vi "Vision_Processing_L_R6.vi"(0 "Current State":T2(ring), 1 "Image Dst":T7=refnum, 2 "Inpute Image":T7=refnum, 3 "Startup Flag":bool, 5 "Current ROI Descriptor":T12={"Global Rectangle"=[81, 70, 256, 199], "Contours"=[{"ID"=enum."External", "Type"=12, "Coordinates"=[81, 70, 256, 199, 0]}]} {"Contours"."Type" items=["No Selection", "Point", "Line", "Rectangle", "Oval", "Polygon", "Freehand Region", "Annulus", "Unused2", "Unused3", "Broken Line", "Freehand Line", "Rotated Rectangle"]}, 7 "error in (no error)":errorcluster, 8 "Current Settings":T10={"Curve Parameters"={"Extraction Mode"=1, "Edge Threshold"=150, "Edge Filter Size"=0, "Min Length"=25, "Row Search Step Size"=15, "Col Search Step Size"=15, "Max Endpoint Gap"=2, "Closed"=TRUE, "Subpixel"=TRUE}, "Match Mode"={"Rotation"=TRUE, "Scale"=TRUE, "Occlusion"=TRUE, "Reserved"=FALSE, "Reserved"=FALSE, "Reserved"=FALSE}, "Range Settings"=[{"Match Constraints"=0, "Min"=-5.0, "Max"=5.0}, {"Match Constraints"=1, "Min"=90.5926284790039, "Max"=120.5926284790039}, {"Match Constraints"=2, "Min"=0.0, "Max"=25.0}], "Number of Matches"=1, "Minimum Match Score"=866.6676, "SubPixel Accuracy"=TRUE, "Adv. Geometric Match Options 2"=[{"Setup Data Item"=20, "Item Value"=0.0}, {"Setup Data Item"=22, "Item Value"=1.0}]} {"Curve Parameters"."Extraction Mode" items=["Normal", "Uniform Regions"]; "Curve Parameters"."Edge Filter Size" items=["Fine", "Normal", "Contour Tracing"]; "Curve Parameters"."Max Endpoint Gap" min=0; "Curve Parameters"."Col Search Step Size" min=1 max=255 step=1; "Curve Parameters"."Row Search Step Size" min=1 max=255 step=1; "Curve Parameters"."Min Length" min=0; "Curve Parameters"."Edge Threshold" min=1 max=350 step=1; "Range Settings"."Max" format="%.2f"; "Range Settings"."Min" format="%.2f"; "Range Settings"."Match Constraints" items=["Rotation Angle (degrees)", "Scale Factor (%)", "Occlusion (%)"]; "Adv. Geometric Match Options 2"."Setup Data Item" items=["Curve Extraction Mode", "Curve Edge Threshold", "Curve Edge Filter Size", "Min Curve Length", "Curve Row Search Step Size", "Curve Col Search Step Size", "Curve Max Endpoint Gap", "Extract Closed Curves", "Enable Subpixel Curve Extraction", "Enable Correlation Score", "Enable Subpixel Accuracy", "Subpixel Iterations", "Subpixel Tolerance", "Initial Match List Length", "Enable Target Template Curve Score", "Min Match Separation Distance", "Min Match Separation Angle", "Min Match Separation Scale", "Max Match Overlap", "Enable Coarse Result", "Enable Calibration Support", "Enable Contrast Reversal", "Search Strategy", "Refinement Match Factor", "Subpixel Match Factor"]}, 9 "Sub Beacon Search Enable":bool[](array[boolean])=[FALSE, FALSE, FALSE, FALSE, FALSE], 10 "History Data - IN":T6={"Valid Beacon History - in"=[TRUE, TRUE, TRUE, TRUE, TRUE, TRUE, TRUE, TRUE, TRUE, TRUE, TRUE, TRUE, TRUE, TRUE, TRUE, TRUE, TRUE, TRUE, TRUE, TRUE], "Valid Score History"=[1000.0, 989.88427734375, 989.88427734375, 989.88427734375, 988.6851196289062, 989.88427734375, 989.0393676757812, 988.6851196289062, 989.88427734375, 987.4860229492188, 989.88427734375, 992.1041870117188, 989.3124389648438, 990.905029296875, 990.5115356445312, 992.1041870117188, 992.1041870117188, 989.88427734375, 991.870361328125, 987.4860229492188], "Valid Scale History"=[103.47016143798828, 106.12324523925781, 106.12324523925781, 106.12324523925781, 106.12324523925781, 106.12324523925781, 106.12324523925781, 106.12324523925781, 106.12324523925781, 106.12324523925781, 106.12324523925781, 105.79054260253906, 106.12324523925781, 105.71609497070312, 106.04004669189453, 105.79054260253906, 105.79054260253906, 106.12324523925781, 105.74315643310547, 106.12324523925781]} {"Valid Scale History" format="%#_13g"; "Valid Score History" format="%#_13g"}, 13 "Last Averages":T1={"Avg Scale - Last"=105.5926284790039, "Avg Score - Last"=991.6675903320313}, 16 "History Size":i32=10, 26 "State Count - in":i32) -> (4 "State Count - out":i32=1, 11 "Avg Scale":dbl=105.5926284790039, 12 "Avg Score":dbl=991.6675903320313, 14 "Tracking Info":T3={"Tracking Coordinates"={"X"=168.53689575195312, "Y"=129.63653564453125}, "Current Valid"=TRUE, "Current State - Out"=enum."Sub - 2"}, 15 "Next Main ROI Descriptor":T4={"Global Rectangle"=[81, 70, 256, 199], "Contours"=[{"ID"=enum."External", "Type"=12, "Coordinates"=[81, 70, 256, 199, 0]}]} {"Contours"."Type" items=["No Selection", "Point", "Line", "Rectangle", "Oval", "Polygon", "Freehand Region", "Annulus", "Unused2", "Unused3", "Broken Line", "Freehand Line", "Rotated Rectangle"]}, 17 "Beacon - Scales":sgl[](array[numeric])=[97.53761, 105.154755, 0.0, 0.0, 0.0], 18 "History Data - Out":T5={"Valid Beacon History\nOut"=[TRUE, TRUE, TRUE, TRUE, TRUE, TRUE, TRUE, TRUE, TRUE, TRUE, TRUE, TRUE, TRUE, TRUE, TRUE, TRUE, TRUE, TRUE, TRUE, TRUE], "Valid Score History\nOut"=[1000.0, 989.88427734375, 989.88427734375, 989.88427734375, 988.6851196289062, 989.88427734375, 989.0393676757812, 988.6851196289062, 989.88427734375, 987.4860229492188, 989.88427734375, 992.1041870117188, 989.3124389648438, 990.905029296875, 990.5115356445312, 992.1041870117188, 992.1041870117188, 989.88427734375, 991.870361328125, 987.4860229492188], "Valid Scale History\nOut"=[103.47016143798828, 106.12324523925781, 106.12324523925781, 106.12324523925781, 106.12324523925781, 106.12324523925781, 106.12324523925781, 106.12324523925781, 106.12324523925781, 106.12324523925781, 106.12324523925781, 105.79054260253906, 106.12324523925781, 105.71609497070312, 106.04004669189453, 105.79054260253906, 105.79054260253906, 106.12324523925781, 105.74315643310547, 106.12324523925781]} {"Valid Scale History\nOut" format="%#_13g"; "Valid Score History\nOut" format="%#_13g"}, 19 "Y Coordinates":sgl[](array[numeric])=[137.61583, 129.42519, 0.0, 0.0, 0.0], 20 "Beacons Found":bool[](array[boolean])=[TRUE, TRUE, FALSE, FALSE, FALSE], 21 "X Coordinates":sgl[](array[numeric])=[137.6292, 203.13261, 0.0, 0.0, 0.0], 22 "Next State":T2(ring), 23 "Lock Status":bool=TRUE, 24 "Startup Flag - out":bool, 25 "New Settings":T10={"Curve Parameters"={"Extraction Mode"=1, "Edge Threshold"=150, "Edge Filter Size"=0, "Min Length"=25, "Row Search Step Size"=15, "Col Search Step Size"=15, "Max Endpoint Gap"=2, "Closed"=TRUE, "Subpixel"=TRUE}, "Match Mode"={"Rotation"=TRUE, "Scale"=TRUE, "Occlusion"=TRUE, "Reserved"=FALSE, "Reserved"=FALSE, "Reserved"=FALSE}, "Range Settings"=[{"Match Constraints"=0, "Min"=-5.0, "Max"=5.0}, {"Match Constraints"=1, "Min"=90.5926284790039, "Max"=120.5926284790039}, {"Match Constraints"=2, "Min"=0.0, "Max"=25.0}], "Number of Matches"=1, "Minimum Match Score"=866.6676, "SubPixel Accuracy"=TRUE, "Adv. Geometric Match Options 2"=[{"Setup Data Item"=20, "Item Value"=0.0}, {"Setup Data Item"=22, "Item Value"=1.0}]} {"Curve Parameters"."Extraction Mode" items=["Normal", "Uniform Regions"]; "Curve Parameters"."Edge Filter Size" items=["Fine", "Normal", "Contour Tracing"]; "Curve Parameters"."Max Endpoint Gap" min=0; "Curve Parameters"."Col Search Step Size" min=1 max=255 step=1; "Curve Parameters"."Row Search Step Size" min=1 max=255 step=1; "Curve Parameters"."Min Length" min=0; "Curve Parameters"."Edge Threshold" min=1 max=350 step=1; "Range Settings"."Max" format="%.2f"; "Range Settings"."Min" format="%.2f"; "Range Settings"."Match Constraints" items=["Rotation Angle (degrees)", "Scale Factor (%)", "Occlusion (%)"]}, 27 "Right Image 2":T7(plugin-control))   [LabVIEW 2015]
uses:
  <vilib>/vision/Image Controls.llb/IMAQ Image.ctl
  <vilib>/vision/Pattern Matching.llb/IMAQ Curve Parameters.ctl
  <vilib>/vision/Pattern Matching.llb/IMAQ Match Range Setting.ctl
panel:
  in  "Sub - 4 - FIle Path":path=path "/home/lvuser/natinst/bin/BeaconTemplates/4_beacons_left.png"
  in  "3 / 2\nTransition Scale":sgl=100.0
  in  "Score\nCushion- tight":dbl=75.0
  in  "Main ROI Decay\nper Fail (Vertical)":i32=5
  in  "ROI_factor(Horiztonal) SCR":sgl=1.7
  in  "ROI_factor(vertical) SCR":sgl=1.5
  in  "Sub - 2 File Path":path=path "/home/lvuser/natinst/bin/BeaconTemplates/2_beacons_left.png"
  in  "Scale Decay \nFactor":dbl=0.5
  in  "Scale Decay \nFactor":dbl=5.0
  in  "Valid Treshold\nfor Lock":i16=3
  in  "Horiztonall Beacon \nCushion (pixels)":sgl=25.0
  out "New Min Score":dbl=866.6675903320313
  out "New Low Scale":dbl=90.5926284790039
  out "New high Scale":dbl=120.5926284790039
  in  "Absolute\nMinimum Score":dbl=700.0
  in  "Absolute\nMaximum Scale":dbl=300.0
  in  "Absolute\nMinimum Scale":dbl=10.0
  in  "Default No Lock\nSetting Values":T11={"Min Scale"=20.0, "Max Scale"=170.0, "Min Score"=800.0}
  in  "Score\nCushion":dbl=125.0
  in  "Scale \nCushion":dbl=15.0
  in  "5 / 4\nTransition Scale":sgl=78.0
  in  "4 / 3\nTransition Scale":sgl=85.0
  in  "Timeout \nThrehsold":i32=1000
  in  "Main ROI Decay\nper Fail (Horiztonal)":i32=25
  in  "ROI_factor(Horiztonal) LR":sgl=5.0
  in  "ROI_factor(vertical) LR":sgl=1.5
  in  "ROI_factor(vertical) SR":sgl=2.7
  in  "ROI_factor(Horiztonal) SR":sgl=2.0
  out "Current  Score":sgl=1000.0
  out "Current  Scale":sgl=103.47016
  in  "Fail Count - In":i32
  in  "Sub Beacon Template File Path - ARRAY":path[](array[path])=[path "/home/lvuser/natinst/bin/BeaconTemplates/Sub1.png", path "/home/lvuser/natinst/bin/BeaconTemplates/Sub2.png", path "/home/lvuser/natinst/bin/BeaconTemplates/Sub3.png", path "/home/lvuser/natinst/bin/BeaconTemplates/Sub4.png", path "/home/lvuser/natinst/bin/BeaconTemplates/Sub5.png"]
  in  "Sub - 3 - FIle Path":path=path "/home/lvuser/natinst/bin/BeaconTemplates/3_beacons_left.png"
  in  "Normal - 5 - File Path":path=path "/home/lvuser/natinst/bin/BeaconTemplates/5_beacons.png"
  # "INPUTS"
  # "FILE PATHS"
  # "CONFIG"
  # "OUTPUTS"
  # "************"
  # "Range"
  # "Range"
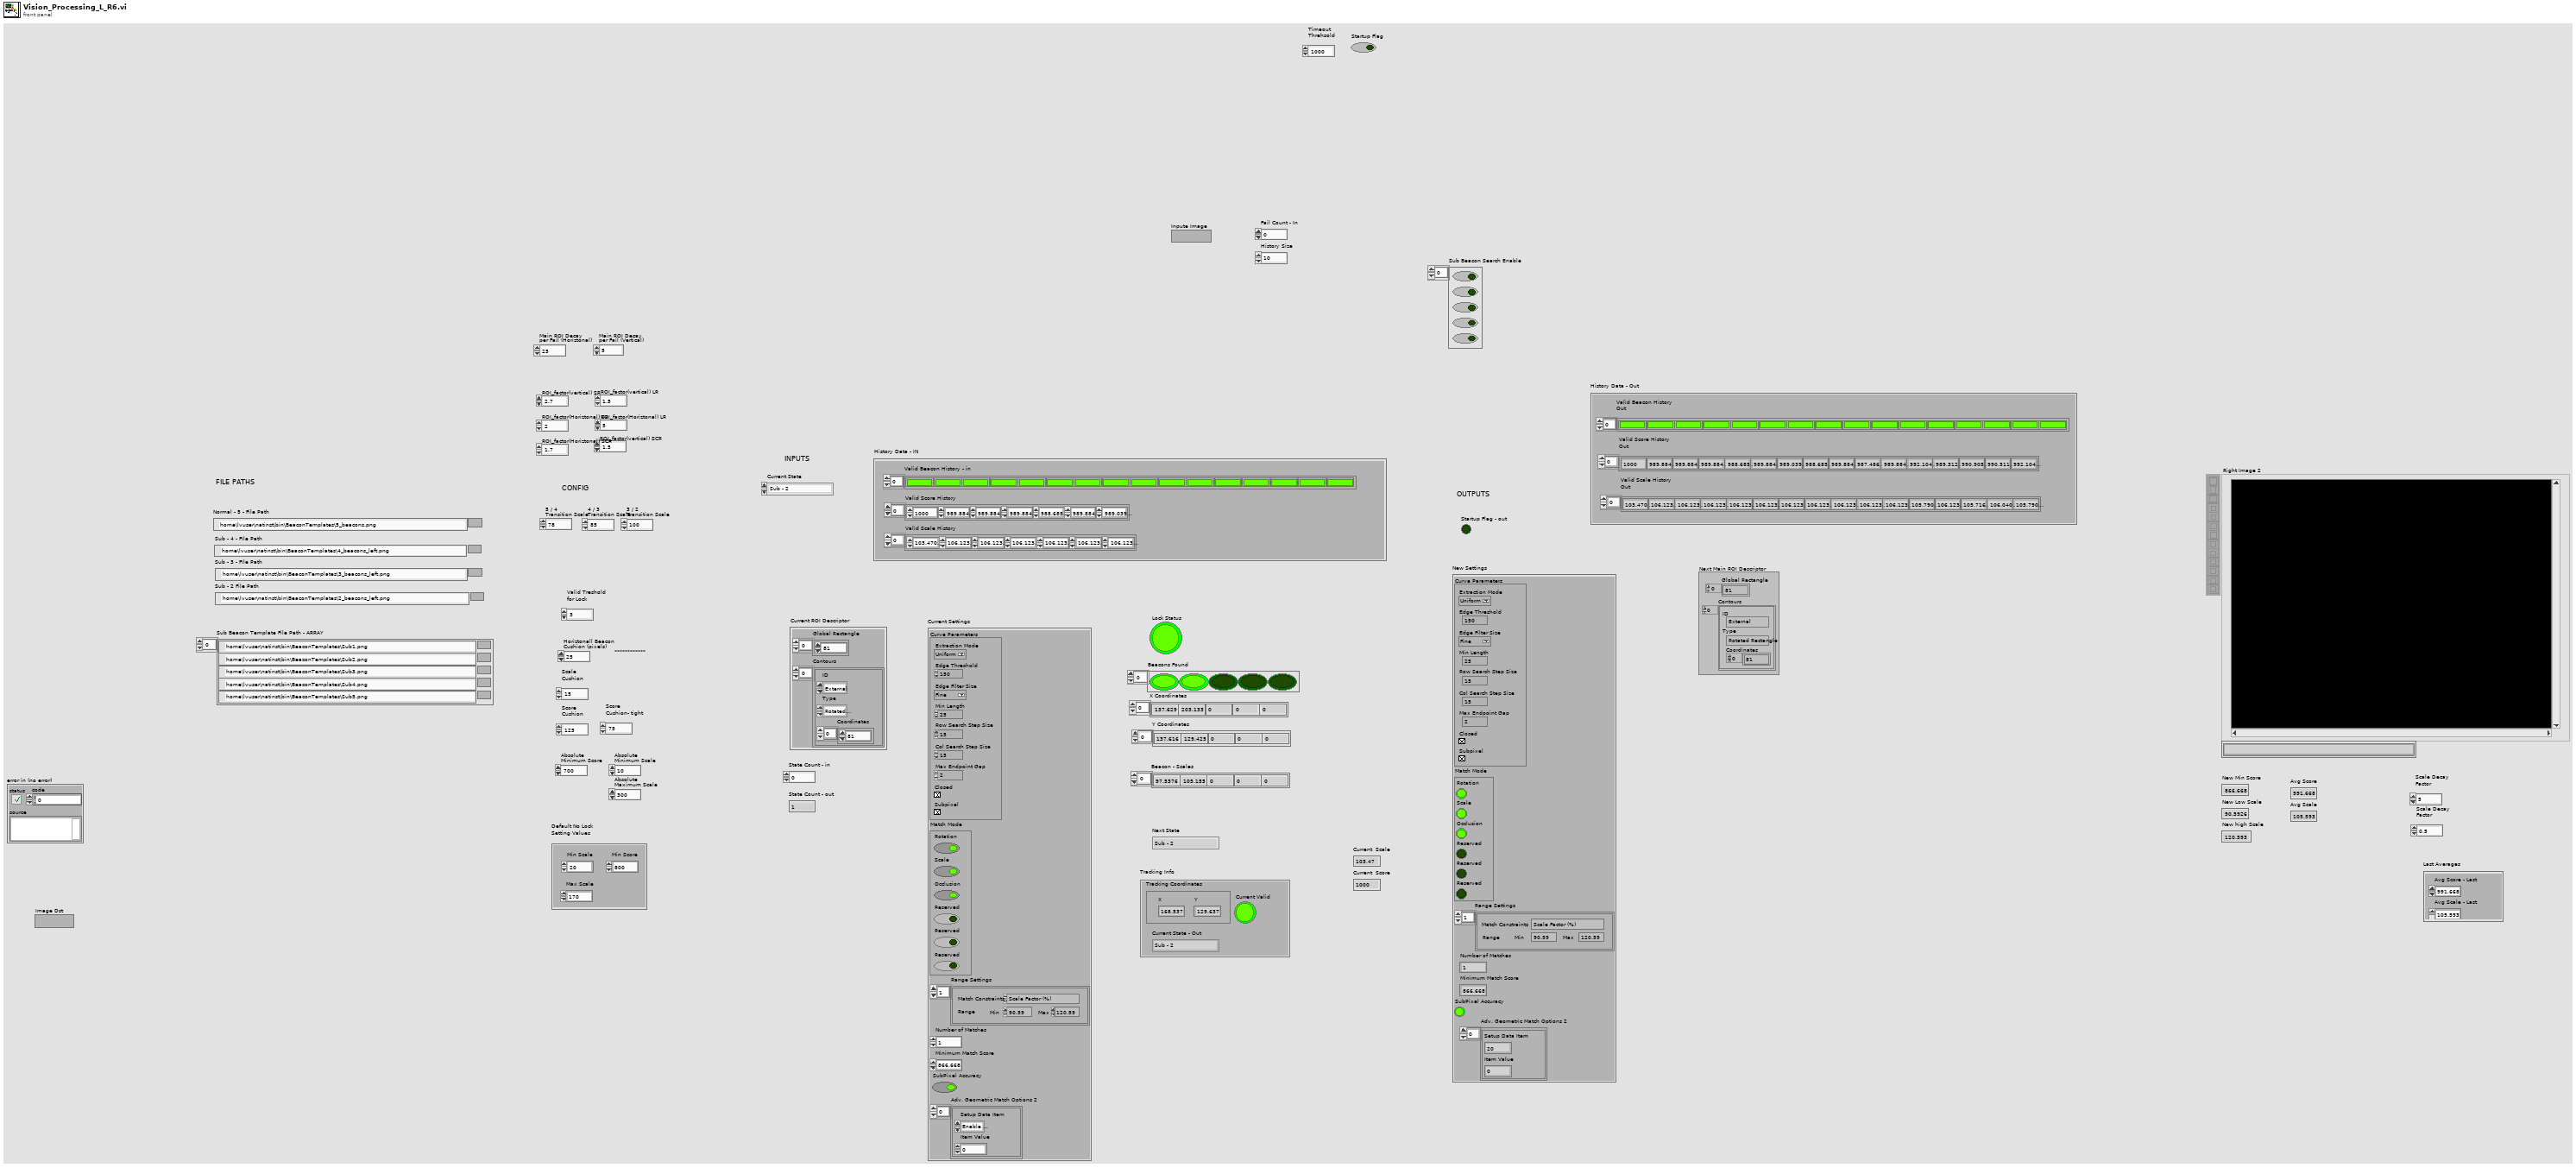
[diagram p1: front panel]
types:
  T1 = cluster{"Avg Scale - Last":dbl, "Avg Score - Last":dbl}
  T2 = enum16{"Sub - 2", "Sub - 3", "Sub - 4", "Normal - 5"}
  T3 = cluster{"Tracking Coordinates":cluster{"X":dbl, "Y":dbl}, "Current Valid":bool, "Current State - Out":enum16{"Sub - 2", "Sub - 3", "Sub - 4", "Normal - 5"}}
  T4 = typedef "ROI Descriptor" = cluster{"Global Rectangle":i32[], "Contours":cluster{"ID":enum32{"External", "Internal"}, "Type":u32, "Coordinates":i32[]}[]}
  T5 = cluster{"Valid Beacon History\nOut":bool[], "Valid Score History\nOut":dbl[], "Valid Scale History\nOut":dbl[]}
  T6 = cluster{"Valid Beacon History - in":bool[], "Valid Score History":dbl[], "Valid Scale History":dbl[]}
  T7 = typedef "IMAQ Image.ctl" = refnum<image>
  T8 = typedef "IMAQ Curve Parameters.ctl" = cluster{"Extraction Mode":u32, "Edge Threshold":i32, "Edge Filter Size":u32, "Min Length":i32, "Row Search Step Size":i32, "Col Search Step Size":i32, "Max Endpoint Gap":i32, "Closed":bool, "Subpixel":bool}
  T9 = typedef "IMAQ Match Range Setting.ctl" = cluster{"Match Constraints":u32, "Min":dbl, "Max":dbl}
  T10 = cluster{"Curve Parameters":T8, "Match Mode":cluster{"Rotation":bool, "Scale":bool, "Occlusion":bool, "Reserved":bool, "Reserved":bool, "Reserved":bool}, "Range Settings":T9[], "Number of Matches":i32, "Minimum Match Score":sgl, "SubPixel Accuracy":bool, "Adv. Geometric Match Options 2":cluster{"Setup Data Item":u16, "Item Value":dbl}[]}
  T11 = cluster{"Min Scale":dbl, "Max Scale":dbl, "Min Score":dbl}
  T12 = cluster{"Global Rectangle":i32[], "Contours":cluster{"ID":enum32{"External", "Internal"}, "Type":u32, "Coordinates":i32[]}[]}
  T13 = typedef "IMAQ GM Match Report.ctl" = cluster{"Position":cluster{"x":sgl, "y":sgl}, "Angle":sgl, "Scale":sgl, "Score":sgl, "Bounding Box":cluster{"x":sgl, "y":sgl}[], "Contrast Reversed":bool, "Occlusion %":sgl, "Template Target Curve Score":sgl, "Target Template Curve Score":sgl, "Correlation Score":sgl}
  T14 = cluster{"Matches (Geometric Matching 1)[0]":T13, "Matches (Geometric Matching 1)[1]":T13, "Matches (Geometric Matching 1)[2]":T13, "Matches (Geometric Matching 1)[3]":T13, "Matches (Geometric Matching 1)[4]":T13, "Matches (Geometric Matching 1)[5]":T13, "Matches (Geometric Matching 1)[6]":T13, "Matches (Geometric Matching 1)[7]":T13, "Matches (Geometric Matching 1)[8]":T13}
  T15 = cluster{"Bounding Box[0]":cluster{"x":sgl, "y":sgl}, "Bounding Box[1]":cluster{"x":sgl, "y":sgl}, "Bounding Box[2]":cluster{"x":sgl, "y":sgl}, "Bounding Box[3]":cluster{"x":sgl, "y":sgl}, "Bounding Box[4]":cluster{"x":sgl, "y":sgl}, "Bounding Box[5]":cluster{"x":sgl, "y":sgl}, "Bounding Box[6]":cluster{"x":sgl, "y":sgl}, "Bounding Box[7]":cluster{"x":sgl, "y":sgl}, "Bounding Box[8]":cluster{"x":sgl, "y":sgl}}
  T16 = cluster{"Position":cluster{"x":sgl, "y":sgl}, bool, "Current State":enum16{"Sub - 2", "Sub - 3", "Sub - 4", "Normal - 5"}}
  T17 = typedef "IMAQ Rectangle" = cluster{"Left":i32, "Top":i32, "Right":i32, "Bottom":i32, "Rotation":dbl}
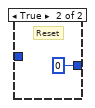
[diagram p2: hidden frame]
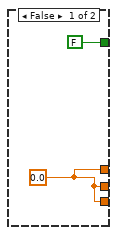
[diagram p3: hidden frame]
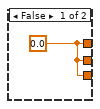
[diagram p4: hidden frame]
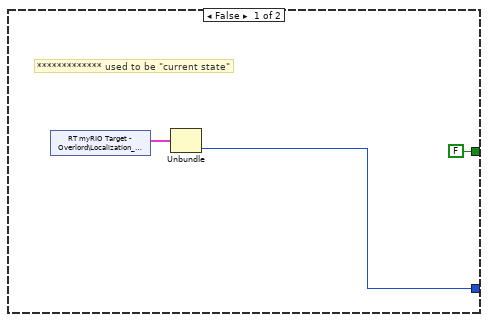
[diagram p8: hidden frame]
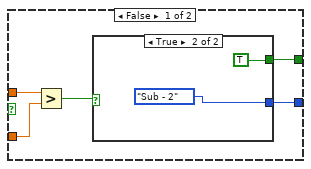
[diagram p9: hidden frame]
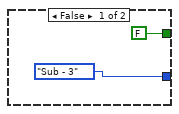
[diagram p10: hidden frame]
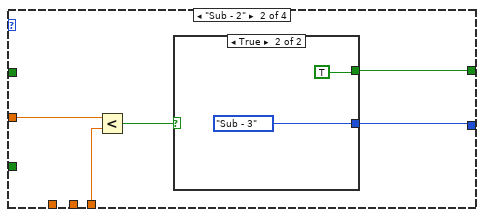
[diagram p11: hidden frame]
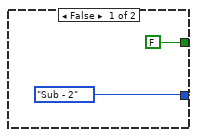
[diagram p12: hidden frame]
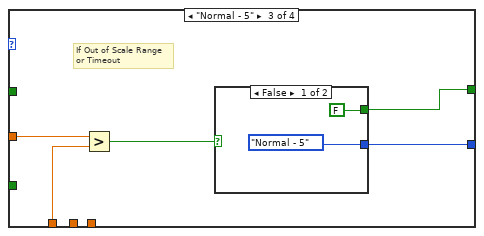
[diagram p13: hidden frame]
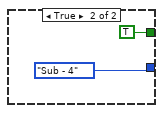
[diagram p14: hidden frame]
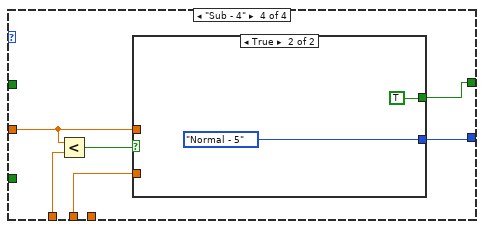
[diagram p15: hidden frame]
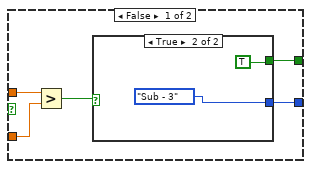
[diagram p16: hidden frame]
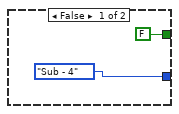
[diagram p17: hidden frame]
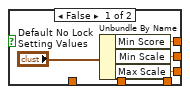
[diagram p19: hidden frame]
diagram:
  (unwired) enum16{"Short Range", "Long Range"}."Short Range"
  # "Next Settings"
  n1 = flat-sequence {
    tunnel: [w8] -> w3
    tunnel: [w7] -> w2
    tunnel: ["Image Dst"] -> w1
    tunnel: w3 -> [w134]
    tunnel: w2 -> [w132]
    tunnel: w1 -> [w133]
    frame #0 {
      # "APPLY FILTERING"
      n2 = call "Camera - Filtering"("Image In"="Inpute Image", "Image Dst"="Image Dst", "error in"="error in (no error)") -> ("Image Out"=w8:T7, "error out"=w7:errorcluster)  [unwired: 23 in]
    }
    frame #1 {
      w93 = u32 1 ("index")
      w114 = u8 5
      # "Transition States (y/n)"
      # "Start up Template"
      # "Image Lock"
      # "Current is Valid"
      # "Update Tracking Coordinates"
      # "CURRENT VALID"
      # "*************"
      # "Beacon - Y"
      # "Beacon - X"
      # "Beacons Found"
      # "Build ROI for Individual Beacons Based on Main Bounding Box"
      # "Starting X Lower Bound"
      # "Length of\nIndividual Beacon ROI"
      # "Length of Bounding Box"
      # "Choose ROI Factor based on Next State"
      # "Current Match"
      # "Current ROI"
      # "Image Lock"
      # "Force SR on Startup"
      # "Valid History"
      # "Draw ROI and stuff on outputi mage"
      # "Pull Down Startup IF Already True and Lock\nOtherwise don't update"
      # "Next Settings"
      # "Apply Limits to Settings"
      # "Scale"
      # "Min Score"
      # "Lower Scale"
      # "Upper Scale"
      # "Current Settings"
      # "Current Min\n& Max Scale"
      # "Current Valid"
      # "Update Search Settings"
      # "Update Template State"
      # "Calculate Average Scale/Score"
      # "max avg"
      # "Min Required to use avarage"
      # "Valid  Ccount\n(up to 3)"
      # "****# of previous in history that must be true\nin order for position to be considered \"locked\""
      # "Update Shift Arrays"
      # "# of Beacons Found to be valid"
      # "# of beacons"
      # "Matches"
      # "image out"
      n3 = Select(t=T2."Normal - 5", s="Startup Flag", f="Current State") -> (s? t:f=w15:T2)
      n4 = case shown="\"Sub - 2\"" w15 {
        tunnel: w134 -> [w443 w475 w506 w541]
        tunnel: w133 -> [w442 w474 w505 w540]
        tunnel: "Current ROI Descriptor" -> [w441 w473 w503 w539]
        tunnel: "Current Settings" -> [w440 w472 w502 w538]
        tunnel: [w436 w468 w499 w534] -> w52
        tunnel: [w435 w467 w500 w533] -> w73
        tunnel: [w433 w465 w501 w531] -> w123
        tunnel: w132 -> [_ _ w504 w530]
        tunnel: "Sub Beacon Search Enable" -> [w434 w466 w507 w529]
        tunnel: [sgl 3.0 ("y") sgl 2.0 ("y") 4.0 sgl 5.0 ("y")] -> w130
        tunnel: [w431 w463 w497 w527] -> w129
        tunnel: [2 1 3 4] -> w124
        frame "Sub - 3" {
          n5 = call "Short Range 2"("Image In"=w443, "Image Dst"=w442, "ROI Descriptor (Geometric Matching 1)"=w441, "Settings (Geometric Matching 1)"=w440, "Template File Path (Geometric Matching 1)"="Sub - 3 - FIle Path") -> ("Image Out"=w435:T7, "Matches (Geometric Matching 1)"=w436:T13[], "Number of Matches (Geometric Matching 1)"=w437:i32, "error out"=w431:errorcluster)  [unwired: 19 in]
          n6 = Equal?(x=w437, y=1) -> (x = y?=w438:bool)
          n7 = case shown="True" w438 {
            tunnel: w434 -> [w451 w454]
            tunnel: [w444 w455] -> w433
            frame False {
              w445 = FALSE
              # "F"
              # "No Main Found,\nDon't Search any Subs"
              n8 = Replace Array Subset(array=w451, new element #1=w445, index #1=0 ("y"), new element #2=w445, index #2=1 ("y"), new element #3=w445, index #3=2 ("y"), new element #4=w445, index #4=3 ("y"), new element #5=w445, index #5=4 ("y")) -> (w444:bool[])
            }
            frame True {
              w453 = TRUE
              w452 = FALSE
              n9 = Replace Array Subset(array=w454, new element #1=w453, index #1=0 ("y"), new element #2=w453, index #2=1 ("y"), new element #3=w453, index #3=2 ("y"), new element #4=w452, index #4=3 ("y"), new element #5=w452, index #5=4 ("y")) -> (w455:bool[])
            }
          }
        }
        frame "Sub - 2" {
          n10 = call "Short Range"("Image In"=w475, "Image Dst"=w474, "ROI Descriptor (Geometric Matching 1)"=w473, "Settings (Geometric Matching 1)"=w472, "Template File Path (Geometric Matching 1)"="Sub - 2 File Path") -> ("Image Out"=w467:T7, "Matches (Geometric Matching 1)"=w468:T13[], "Number of Matches (Geometric Matching 1)"=w469:i32, "error out"=w463:errorcluster)  [unwired: 19 in]
          n11 = Equal?(x=w469, y=1) -> (x = y?=w470:bool)
          n12 = case shown="True" w470 {
            tunnel: w466 -> [w483 w486]
            tunnel: [w476 w487] -> w465
            frame False {
              w477 = FALSE
              # "F"
              # "No Main Found,\nDon't Search any Subs"
              n13 = Replace Array Subset(array=w483, new element #1=w477, index #1=0 ("y"), new element #2=w477, index #2=1 ("y"), new element #3=w477, index #3=2 ("y"), new element #4=w477, index #4=3 ("y"), new element #5=w477, index #5=4 ("y")) -> (w476:bool[])
            }
            frame True {
              w485 = TRUE
              w484 = FALSE
              # "Search for specific Beacons"
              n14 = Replace Array Subset(array=w486, new element #1=w485, index #1=0 ("y"), new element #2=w485, index #2=1 ("y"), new element #3=w484, index #3=2 ("y"), new element #4=w484, index #4=3 ("y"), new element #5=w484, index #5=4 ("y")) -> (w487:bool[])
            }
          }
        }
        frame "Sub - 4" {
          # "**Make sure this selects the \nappropriate beacons to search for!!"
          n15 = call "Dumping Range"("Image In"=w506, "Image Dst"=w505, "ROI Descriptor (Geometric Matching 1)"=w503, "Settings (Geometric Matching 1)"=w502, "Template File Path (Geometric Matching 1)"="Sub - 4 - FIle Path", "error in"=w504) -> ("Image Out"=w500:T7, "Matches (Geometric Matching 1)"=w499:T13[], "Number of Matches (Geometric Matching 1)"=w496:i32, "error out"=w497:errorcluster)  [unwired: 18 in]
          n16 = Equal?(x=w496, y=1) -> (x = y?=w494:bool)
          n17 = case shown="True" w494 {
            tunnel: w507 -> [w516 w519]
            tunnel: [w509 w520] -> w501
            frame False {
              w510 = FALSE
              # "F"
              # "No Main Found,\nDon't Search any Subs"
              n18 = Replace Array Subset(array=w516, new element #1=w510, index #1=0 ("y"), new element #2=w510, index #2=1 ("y"), new element #3=w510, index #3=2 ("y"), new element #4=w510, index #4=3 ("y"), new element #5=w510, index #5=4 ("y")) -> (w509:bool[])
            }
            frame True {
              w517 = TRUE
              n19 = Replace Array Subset(array=w519, new element #1=w517, index #1=0 ("y"), new element #2=w517, index #2=1 ("y"), new element #3=w517, index #3=2 ("y"), new element #4=w517, index #4=3 ("y"), new element #5=FALSE, index #5=4 ("y")) -> (w520:bool[])
            }
          }
        }
        frame "Normal - 5" {
          n20 = call "Long Range"("Image In"=w541, "Image Dst"=w540, "ROI Descriptor (Geometric Matching 1)"=w539, "Settings (Geometric Matching 1)"=w538, "Template File Path (Geometric Matching 1)"="Normal - 5 - File Path", "error in"=w530) -> ("Image Out"=w533:T7, "Matches (Geometric Matching 1)"=w534:T13[], "Number of Matches (Geometric Matching 1)"=w536:i32, "error out"=w527:errorcluster)  [unwired: 18 in]
          n21 = Equal?(x=w536, y=1) -> (x = y?=w532:bool)
          n22 = case shown="True" w532 {
            tunnel: w529 -> [w549 w551]
            tunnel: [w542 w550] -> w531
            frame False {
              w543 = FALSE
              # "F"
              # "No Main Found,\nDon't Search any Subs"
              n23 = Replace Array Subset(array=w549, new element #1=w543, index #1=0 ("y"), new element #2=w543, index #2=1 ("y"), new element #3=w543, index #3=2 ("y"), new element #4=w543, index #4=3 ("y"), new element #5=w543, index #5=4 ("y")) -> (w542:bool[])
            }
            frame True {
              w552 = TRUE
              # "T"
              # "Search for ALL Beacons"
              n24 = Replace Array Subset(array=w551, new element #1=w552, index #1=0 ("y"), new element #2=w552, index #2=1 ("y"), new element #3=w552, index #3=2 ("y"), new element #4=w552, index #4=3 ("y"), new element #5=w552, index #5=4 ("y")) -> (w550:bool[])
            }
          }
        }
      }
      n25 = Array To Cluster(array=w52) -> (cluster=w42:T14)
      n26 = Unbundle By Name(w42) -> ("Matches (Geometric Matching 1)[0].Position"=w17:cluster{"x":sgl, "y":sgl}, "Matches (Geometric Matching 1)[0].Bounding Box"=w40:cluster{"x":sgl, "y":sgl}[], "Matches (Geometric Matching 1)[0].Scale"=w72:sgl, "Matches (Geometric Matching 1)[0].Score"=w84:sgl)
      "Current  Scale" <- w72
      "Current  Score" <- w84
      n27 = Array To Cluster(array=w40) -> (cluster=w41:T15)
      n28 = Unbundle By Name(w41) -> ("Bounding Box[0].x"=w31:sgl, "Bounding Box[0].y"=w30:sgl, "Bounding Box[2].x"=w29:sgl, "Bounding Box[2].y"=w28:sgl)
      n29 = Bundle("x"=w31, "y"=w30, "x"=w29, "y"=w28) -> (w26:cluster{"x":sgl, "y":sgl, "x":sgl, "y":sgl})  [unwired: 1 in]
      n30 = call "IMAQ Overlay Rectangle"("Rectangle"=w26, "Image"=w73) -> ("Image Out"=w27:T7)  [unwired: 8 in, 1 out]
      n31 = Subtract(x=w29, y=w31) -> (x-y=w35:sgl)
      n32 = Divide(x=w35, y=w130) -> (x/y=w37:dbl)
      n33 = Multiply(x="Horiztonall Beacon \nCushion (pixels)", y=w72) -> (x*y=w25:sgl)
      n34 = Divide(x=w25, y=sgl 100.0) -> (x/y=w22:sgl)
      n35 = Subtract(x=w30, y=w22) -> (x-y=w38:sgl)
      n36 = Add(x=w22, y=w28) -> (x+y=w39:sgl)
      n37 = for {
        N: 5 -> [_]
        tunnel: w123 -> [w180] mode=indexing
        shift-right: [w174] -> _
        shift-left: w31 -> [w179]
        tunnel: w37 -> [w178]
        tunnel: w38 -> [w171]
        tunnel: w39 -> [w170]
        tunnel: [w177] -> w33 mode=indexing
        tunnel: w22 -> [w172]
        # "Divide Bounding Box"
        # "Upper Bound of Current is\nLower Bound for Next"
        n38 = case shown="True" w180 {
          tunnel: w179 -> [w181 w182]
          tunnel: w178 -> [_ w184]
          tunnel: [w181 w183] -> w174
          tunnel: [w181 w182] -> w176
          frame False {
            # "Don't Care"
          }
          frame True {
            # "X Lower Bound"
            n39 = Add(x=w182, y=w184) -> (x+y=w183:dbl)
          }
        }
        n40 = Subtract(x=w176, y=w172) -> (x-y=w175:dbl)
        n41 = Add(x=w174, y=w172) -> (x+y=w173:dbl)
        n42 = call "Bound_RO_R_R0I.vi"("Bottom Right - Y"=w170, "Right - X"=w173, "Top Left - Y"=w171, "Top  Left - x"=w175) -> ("ROI Descriptor"=w177:T4)  [unwired: 7 in]
      }
      n43 = for {
        N: 5 -> [_]
        tunnel: w73 -> [w149]
        tunnel: w129 -> [w148]
        tunnel: w33 -> [w141] mode=indexing
        tunnel: "Sub Beacon Template File Path - ARRAY" -> [w147] mode=indexing
        tunnel: [w146] -> w128 mode=indexing
        tunnel: [w145] -> w127 mode=indexing
        tunnel: [w144] -> w115 mode=indexing
        tunnel: w123 -> [w143] mode=indexing
        tunnel: "Current Settings" -> [w142]
        shift-right: [w139] -> w74
        shift-left: w27 -> [w140]
        tunnel: [w138] -> w63 mode=indexing
        n44 = case shown="True" w143 {
          tunnel: w149 -> [_ w163]
          tunnel: w148 -> [_ w162]
          tunnel: w141 -> [_ w161]
          tunnel: w147 -> [_ w160]
          tunnel: [w150 w156] -> w146
          tunnel: [w150 w155] -> w145
          tunnel: [FALSE w154] -> w144
          tunnel: w142 -> [_ w153]
          tunnel: [w150 w152] -> w138
          frame False {
            w150 = sgl 0.0 ("x")
          }
          frame True {
            n45 = call "Sub Beacon Pattern Match"("Image In"=w163, "ROI Descriptor (Geometric Matching 1)"=w161, "Settings (Geometric Matching 1)"=w153, "Template File Path (Geometric Matching 1)"=w160, "error in"=w162) -> ("Matches (Geometric Matching 1)"=w157:T13[], "Number of Matches (Geometric Matching 1)"=w158:i32)  [unwired: 19 in, 2 out]
            n46 = Equal?(x=w158, y=1) -> (x = y?=w154:bool)
            n47 = case shown="True" w154 {
              tunnel: w157 -> [_ w168]
              tunnel: [w164 w167] -> w156
              tunnel: [w164 w166] -> w155
              tunnel: [w164 w165] -> w152
              frame False {
                w164 = sgl 0.0 ("x")
              }
              frame True {
                n48 = Array To Cluster(array=w168) -> (cluster=w169:T14)
                n49 = Unbundle By Name(w169) -> ("Matches (Geometric Matching 1)[0].Position.x"=w167:sgl, "Matches (Geometric Matching 1)[0].Position.y"=w166:sgl, "Matches (Geometric Matching 1)[0].Scale"=w165:sgl)
              }
            }
          }
        }
        n50 = call "IMAQ Overlay ROI"("ROI Descriptor"=w141, "Image"=w140) -> ("Image Out"=w139:T7)  [unwired: 8 in, 1 out]
      }
      "Beacons Found" <- w115
      "X Coordinates" <- w128
      "Y Coordinates" <- w127
      "Beacon - Scales" <- w63
      n51 = Boolean To (0,1)(Boolean=w115) -> (0, 1=w125:i16[])
      n52 = Add Array Elements(numeric array=w125) -> (sum=w126:i16)
      n53 = Greater Or Equal?(x=w126, y=w124) -> (x >= y?=w16:bool)
      n54 = case shown="False" w16 {
        tunnel: "Fail Count - In" -> [w427 _]
        tunnel: [w426 u16 0] -> w107
        frame False {
          n55 = Increment(x=w427) -> (x+1=w426:i32)
        }
        frame True {
          # "reset fail count"
        }
      }
      n56 = Unbundle By Name("History Data - IN") -> ("Valid Beacon History - in"=w70:bool[], "Valid Score History"=w69:dbl[], "Valid Scale History"=w68:dbl[])
      n57 = Greater?(x=w107, y="Timeout \nThrehsold") -> (0:w19:bool)
      n58 = Decrement(x="History Size") -> (x-1=w121:i32)
      n59 = for {
        N: "History Size" -> [_]
        shift-right: [w404] -> w67
        shift-left: w70 -> [w392]
        tunnel: w121 -> [w400]
        shift-right: [w397] -> w66
        shift-left: w69 -> [w399]
        shift-right: [w396] -> w65
        shift-left: w68 -> [w398]
        tunnel: w84 -> [w395]
        tunnel: w72 -> [w394]
        tunnel: w16 -> [w393]
        i -> [w403]
        # "Reverse Index"
        n60 = Subtract(x=w400, y=w403) -> (x-y=w401:i32)
        n61 = Equal To 0?(x=w401) -> (x = 0?=w402:bool)
        n62 = case shown="True" w402 {
          tunnel: w401 -> [w405 w424]
          tunnel: w392 -> [w415 w417]
          tunnel: [w413 w416] -> w404
          tunnel: w393 -> [_ w425]
          tunnel: w399 -> [w410 w423]
          tunnel: w398 -> [w409 w422]
          tunnel: [w408 w420] -> w397
          tunnel: [w407 w421] -> w396
          tunnel: w395 -> [_ w419]
          tunnel: w394 -> [_ w418]
          frame False {
            # "Shift Old"
            n63 = Decrement(x=w405) -> (x-1=w406:i32)
            n64 = Index Array(array=w415, index=w406) -> (element=w414:bool)
            n65 = Index Array(array=w410, index=w406) -> (element=w412:dbl)
            n66 = Index Array(array=w409, index=w406) -> (element=w411:dbl)
            n67 = Replace Array Subset(array=w415, new element=w414, index=w405) -> (w413:bool[])
            n68 = Replace Array Subset(array=w410, new element=w412, index=w405) -> (w408:dbl[])
            n69 = Replace Array Subset(array=w409, new element=w411, index=w405) -> (w407:dbl[])
          }
          frame True {
            # "Scale"
            # "Score"
            # "Valid"
            # "insert New"
            n70 = Replace Array Subset(array=w423, new element=w419, index=w424) -> (w420:dbl[])
            n71 = Replace Array Subset(array=w422, new element=w418, index=w424) -> (w421:dbl[])
            n72 = Replace Array Subset(array=w417, new element=w425, index=w424) -> (w416:bool[])
          }
        }
      }
      n73 = Boolean To (0,1)(Boolean=w67) -> (0, 1=w119:i16[])
      n74 = Bundle("Valid Beacon History - in"=w67, "Valid Score History"=w66, "Valid Scale History"=w65) -> (→"History Data - Out":T6)  [unwired: 1 in]
      n75 = Add Array Elements(numeric array=w119) -> (sum=w120:i16)
      n76 = Greater Or Equal?(x=w120, y="Valid Treshold\nfor Lock") -> (x >= y?=w85:bool)
      "Lock Status" <- w85
      n77 = Initialize Array(u8 0, w114) -> (w117:u8[])
      n78 = while {
        shift-right: [w375] -> w112
        shift-left: w117 -> [w377]
        tunnel: w67 -> [w383] mode=indexing
        shift-right: [w381] -> w110
        shift-left: u8 0 -> [w384]
        tunnel: "History Size" -> [w382]
        tunnel: w114 -> [w374]
        i -> [w376]
        stop <- w378 stop-if-true
        # "Grab Last 2 Valid Indexes"
        n79 = case shown="True" w383 {
          tunnel: w384 -> [w386 w388]
          tunnel: [w386 w391] -> w381
          tunnel: w377 -> [w385 w390]
          tunnel: w376 -> [_ w389]
          tunnel: [w385 w387] -> w375
          frame False {
          }
          frame True {
            # "Update Index\nto use"
            # "Increment\nValid Count"
            n80 = Replace Array Subset(array=w390, new element=w389, index=w388) -> (w387:u8[])
            n81 = Increment(x=w388) -> (x+1=w391:u8)
          }
        }
        n82 = Greater?(x=w376, y=w382) -> (0:w379:bool)
        n83 = Greater Or Equal?(x=w381, y=w374) -> (x >= y?=w380:bool)
        n84 = Or(x=w380, y=w379) -> (x .or. y?=w378:bool)
      }
      n85 = Greater?(x=w110, y=u8 2) -> (0:w111:bool)
      n86 = case shown="True" w111 {
        tunnel: w110 -> [_ w358]
        tunnel: w112 -> [_ w364]
        tunnel: w66 -> [_ w363]
        tunnel: w65 -> [_ w362]
        tunnel: [w353 w356] -> w81
        tunnel: [w352 w355] -> w82
        frame False {
          n87 = Unbundle("Last Averages") -> ("Avg Scale - Last"=w352:dbl, "Avg Score - Last"=w353:dbl)
        }
        frame True {
          w361 = 0.0
          n88 = for {
            N: w358 -> [_]
            tunnel: w364 -> [w371] mode=indexing
            tunnel: w363 -> [w373]
            tunnel: w362 -> [w372]
            shift-right: [w369] -> w360
            shift-left: w361 -> [w367]
            shift-right: [w370] -> w359
            shift-left: w361 -> [w366]
            # "Fetch Last Valid Values"
            n89 = Index Array(array=w373, index=w371) -> (element=w368:dbl)
            n90 = Index Array(array=w372, index=w371) -> (element=w365:dbl)
            n91 = Add(x=w368, y=w367) -> (x+y=w369:dbl)
            n92 = Add(x=w365, y=w366) -> (x+y=w370:dbl)
          }
          n93 = To Double Precision Float(number=w358) -> (double precision float=w357:dbl)
          n94 = Divide(x=w360, y=w357) -> (x/y=w356:dbl)
          n95 = Divide(x=w359, y=w357) -> (x/y=w355:dbl)
        }
      }
      "Avg Score" <- w81
      "Avg Scale" <- w82
      n96 = Bundle("Position"=w17, w16, "Current State"=w15) -> (→"Tracking Info":T16)  [unwired: 1 in]
      n97 = case shown="True" w85 {
        tunnel: w19 -> [_ w201]
        tunnel: "4 / 3\nTransition Scale" -> [_ w200]
        tunnel: "5 / 4\nTransition Scale" -> [_ w199]
        tunnel: w82 -> [_ w198]
        tunnel: w85 -> [_ w197]
        tunnel: [w191 w196] -> w13
        tunnel: "3 / 2\nTransition Scale" -> [_ w195]
        tunnel: [FALSE w194] -> w11
        frame False {
          # "************* used to be \"current state\""
          n98 = shared-variable "RT myRIO Target - Overlord\\Localization_Variables_r0.lvlib\\Info - Right"() -> (w192:T3)  [unwired: 1 in, 1 out]
          n99 = Unbundle(w192) -> ("Current State - Out"=w191:T2)  [unwired: 2 out]
        }
        frame True {
          # "Timeout"
          n100 = local read "Current State"() -> (w202:T2)
          n101 = case shown="\"Sub - 3\", Default" w202 {
            tunnel: w197 -> [_ _ _ _]
            tunnel: w198 -> [w207 w224 w232 w241]
            tunnel: w201 -> [_ _ _ _]
            tunnel: w200 -> [w208 _ _ w240]
            tunnel: w199 -> [_ _ w231 w243]
            tunnel: [w204 w221 w230 w239] -> w196
            tunnel: w195 -> [w205 w223 _ _]
            tunnel: [w203 w220 w229 w238] -> w194
            frame "Sub - 3", Default {
              n102 = Less?(x=w207, y=w208) -> (x < y?=w206:bool)
              n103 = case shown="True" w206 {
                tunnel: w207 -> [w213 _]
                tunnel: [w210 T2."Sub - 4"] -> w204
                tunnel: w205 -> [w212 _]
                tunnel: [w209 TRUE] -> w203
                frame False {
                  n104 = Greater?(x=w213, y=w212) -> (0:w211:bool)
                  n105 = case shown="True" w211 {
                    tunnel: [T2."Sub - 3" T2."Sub - 2"] -> w210
                    tunnel: [FALSE TRUE] -> w209
                    frame False {
                    }
                    frame True {
                    }
                  }
                }
                frame True {
                }
              }
            }
            frame "Sub - 2" {
              n106 = Less?(x=w224, y=w223) -> (x < y?=w222:bool)
              n107 = case shown="True" w222 {
                tunnel: [T2."Sub - 2" T2."Sub - 3"] -> w221
                tunnel: [FALSE TRUE] -> w220
                frame False {
                }
                frame True {
                }
              }
            }
            frame "Normal - 5" {
              # "If Out of Scale Range\nor Timeout"
              n108 = Greater?(x=w232, y=w231) -> (0:w233:bool)
              n109 = case shown="False" w233 {
                tunnel: [T2."Normal - 5" T2."Sub - 4"] -> w230
                tunnel: [FALSE TRUE] -> w229
                frame False {
                }
                frame True {
                }
              }
            }
            frame "Sub - 4" {
              n110 = Less?(x=w241, y=w243) -> (x < y?=w242:bool)
              n111 = case shown="True" w242 {
                tunnel: w241 -> [w248 _]
                tunnel: [w245 T2."Normal - 5"] -> w239
                tunnel: w240 -> [w247 _]
                tunnel: [w244 TRUE] -> w238
                frame False {
                  n112 = Greater?(x=w248, y=w247) -> (0:w246:bool)
                  n113 = case shown="True" w246 {
                    tunnel: [T2."Sub - 4" T2."Sub - 3"] -> w245
                    tunnel: [FALSE TRUE] -> w244
                    frame False {
                    }
                    frame True {
                    }
                  }
                }
                frame True {
                }
              }
            }
          }
        }
      }
      "Next State" <- w13
      n114 = case shown="False" w11 {
        tunnel: "State Count - in" -> [w136 _]
        tunnel: [w135 0] -> w9
        frame False {
          n115 = Increment(x=w136) -> (x+1=w135:i32)
        }
        frame True {
          # "Reset"
        }
      }
      "State Count - out" <- w9
      n116 = Unbundle By Name("Current Settings") -> ("Minimum Match Score"=w104:sgl, "Range Settings"=w90:T9[])
      n117 = case shown="\"Sub - 4\", Default" w13 {
        tunnel: "ROI_factor(vertical) SR" -> [_ _ w190]
        tunnel: "ROI_factor(Horiztonal) SR" -> [_ _ w189]
        tunnel: "ROI_factor(vertical) LR" -> [_ w188 _]
        tunnel: "ROI_factor(Horiztonal) LR" -> [_ w187 _]
        tunnel: "ROI_factor(vertical) SCR" -> [w186 _ _]
        tunnel: "ROI_factor(Horiztonal) SCR" -> [w185 _ _]
        tunnel: [w186 w188 w190] -> w45
        tunnel: [w185 w187 w189] -> w44
        frame "Sub - 2" {
        }
        frame "Sub - 4", Default {
        }
        frame "Sub - 3" {
        }
      }
      n118 = Index Array(array=w90, index=u32 1) -> (element=w103:T9)
      n119 = Unbundle(w103) -> ("Min"=w101:dbl, "Max"=w100:dbl)  [unwired: 1 out]
      n120 = case shown="False" w85 {
        tunnel: w16 -> [_ w309]
        tunnel: w81 -> [w272 w308]
        tunnel: w82 -> [w271 w307]
        tunnel: w104 -> [w257 w306]
        tunnel: w101 -> [w258 w305]
        tunnel: w100 -> [w259 w304]
        tunnel: [w270 w295] -> w91
        tunnel: [w269 w294] -> w56
        tunnel: [w268 w293] -> w57
        tunnel: "Scale \nCushion" -> [w274 w303]
        tunnel: "Score\nCushion" -> [w273 w302]
        tunnel: "Scale Decay \nFactor" -> [_ w301]
        tunnel: "Scale Decay \nFactor" -> [_ w300]
        tunnel: "Current ROI Descriptor" -> [_ w296]
        tunnel: w52 -> [_ w297]
        tunnel: w45 -> [_ w299]
        tunnel: w44 -> [_ w298]
        tunnel: [w261 w292] -> w43
        frame False {
          # "Initial ROI Descriptor"
          # "Apply No Lock Default for each Template"
          n121 = local read "Startup Flag"() -> (w260:bool)
          n122 = case shown="True" w260 {
            tunnel: [w277 w279] -> w270
            tunnel: [w276 w281] -> w269
            tunnel: [w275 w280] -> w268
            tunnel: w259 -> [_ w280]
            tunnel: w258 -> [_ w281]
            tunnel: w257 -> [_ w279]
            frame False {
              n123 = Unbundle By Name("Default No Lock\nSetting Values") -> ("Min Score"=w277:dbl, "Min Scale"=w276:dbl, "Max Scale"=w275:dbl)
            }
            frame True {
            }
          }
          n124 = disable-structure shown="Disabled" {
            disable-tunnel: [w287 _] -> _
            disable-tunnel: [w286 _] -> _
            disable-tunnel: w274 -> [w285 _]
            disable-tunnel: w273 -> [w284 _]
            disable-tunnel: w272 -> [w283 _]
            disable-tunnel: w271 -> [w282 _]
            frame Disabled {
              n125 = Subtract(x=w283, y=w284) -> ()  [unwired: 1 out]
              n126 = Subtract(x=w282, y=w285) -> (x-y=w287:dbl)
              n127 = Add(x=w285, y=w282) -> (x+y=w286:dbl)
            }
            frame Enabled {
            }
          }
          n128 = Bundle(0, 0, 640, 480, 0) -> (w267:cluster{i32, i32, i32, i32, i32})  [unwired: 1 in]
          n129 = call "IMAQ Convert Rectangle to ROI"("Rectangle"=w267) -> ("ROI Descriptor"=w261:T4)  [unwired: 8 in, 1 out]
        }
        frame True {
          # "Apply Limits to ROI"
          n130 = case shown="True" w309 {
            tunnel: w308 -> [_ w351]
            tunnel: [w324 w347] -> w295
            tunnel: w307 -> [_ w350]
            tunnel: [w323 w346] -> w294
            tunnel: [w322 w345] -> w293
            tunnel: w305 -> [w329 _]
            tunnel: w304 -> [w328 _]
            tunnel: w306 -> [w327 _]
            tunnel: w303 -> [_ w349]
            tunnel: w302 -> [_ w348]
            tunnel: w301 -> [w326 _]
            tunnel: w300 -> [w325 _]
            tunnel: w299 -> [_ w336]
            tunnel: w298 -> [_ w335]
            tunnel: w297 -> [_ w334]
            tunnel: [w313 w333] -> w291
            tunnel: [w312 w332] -> w290
            tunnel: [w311 w331] -> w289
            tunnel: [w310 w330] -> w288
            tunnel: w296 -> [w320 _]
            frame False {
              # "Decrement Score by"
              n131 = Subtract(x=w329, y=w325) -> (x-y=w323:dbl)
              n132 = Add(x=w325, y=w328) -> (x+y=w322:dbl)
              n133 = Subtract(x=w327, y=w326) -> (x-y=w324:dbl)
              n134 = call "IMAQ Convert ROI to Rectangle"("ROI Descriptor"=w320) -> ("Rectangle"=w321:T17)  [unwired: 8 in, 1 out]
              n135 = Unbundle By Name(w321) -> ("Left"=w317:i32, "Top"=w316:i32, "Right"=w315:i32, "Bottom"=w314:i32)
              n136 = Subtract(x=w317, y="Main ROI Decay\nper Fail (Horiztonal)") -> (x-y=w313:i32)
              n137 = Add(x=w315, y="Main ROI Decay\nper Fail (Horiztonal)") -> (x+y=w311:i32)
              n138 = Add(x=w314, y="Main ROI Decay\nper Fail (Vertical)") -> (x+y=w310:i32)
              n139 = Subtract(x=w316, y="Main ROI Decay\nper Fail (Vertical)") -> (x-y=w312:i32)
            }
            frame True {
              # "Scale / Score"
              # "Main ROI"
              # "Horizontal Scale \n(smaller number = smaller ROI)"
              n140 = Subtract(x=w351, y=w348) -> (x-y=w347:dbl)
              n141 = Subtract(x=w350, y=w349) -> (x-y=w346:dbl)
              n142 = Add(x=w349, y=w350) -> (x+y=w345:dbl)
              n143 = Array To Cluster(array=w334) -> (cluster=w344:T14)
              n144 = Unbundle By Name(w344) -> ("Matches (Geometric Matching 1)[0].Position.x"=w338:sgl, "Matches (Geometric Matching 1)[0].Position.y"=w340:sgl, "Matches (Geometric Matching 1)[0].Scale"=w339:sgl)
              n145 = Divide(x=w339, y=w336) -> (x/y=w341:sgl)
              n146 = Multiply(x=w339, y=w335) -> (x*y=w343:sgl)
              n147 = Divide(x=w343, y=sgl 2.0) -> (x/y=w337:sgl)
              n148 = Add(x=w340, y=w341) -> (x+y=w330:sgl)
              n149 = Subtract(x=w340, y=w341) -> (x-y=w332:sgl)
              n150 = Subtract(x=w338, y=w337) -> (x-y=w333:sgl)
              n151 = Add(x=w337, y=w338) -> (x+y=w331:sgl)
            }
          }
          n152 = call "Bound_RO_L_R0I.vi"("Bottom Right - Y"=w288, "Right - X"=w289, "Top Left - Y"=w290, "Top  Left - x"=w291) -> ("ROI Descriptor"=w292:T4)  [unwired: 7 in]
        }
      }
      "Next Main ROI Descriptor" <- w43
      n153 = And(x="Startup Flag", y=w85) -> (x .and. y?=w88:bool)
      n154 = case shown="True" w88 {
        tunnel: "Startup Flag" -> [w255 _]
        tunnel: [w255 FALSE] -> w87
        frame False {
        }
        frame True {
        }
      }
      "Startup Flag - out" <- w87
      n155 = Less?(x=w91, y="Absolute\nMinimum Score") -> (x < y?=w95:bool)
      n156 = Less?(x=w56, y="Absolute\nMinimum Scale") -> (x < y?=w59:bool)
      n157 = Greater?(x=w57, y="Absolute\nMaximum Scale") -> (0:w54:bool)
      n158 = Greater?(x=w56, y=w57) -> (0:w60:bool)
      n159 = Less?(x=w57, y=w56) -> (x < y?=w55:bool)
      n160 = Select(t="Absolute\nMinimum Score", s=w95, f=w91) -> (s? t:f=w97:dbl)
      "New Min Score" <- w97
      n161 = Or(x=w59, y=w60) -> (x .or. y?=w61:bool)
      n162 = Or(x=w54, y=w55) -> (x .or. y?=w58:bool)
      n163 = Select(t="Absolute\nMinimum Scale", s=w61, f=w56) -> (s? t:f=w75:dbl)
      "New Low Scale" <- w75
      n164 = Select(t="Absolute\nMaximum Scale", s=w58, f=w57) -> (s? t:f=w76:dbl)
      "New high Scale" <- w76
      n165 = Bundle("index"=w93, "Min"=w75, "Max"=w76) -> (w92:cluster{"index":u32, "Min":dbl, "Max":dbl})  [unwired: 1 in]
      n166 = Replace Array Subset(array=w90, new element=w92, index=w93) -> (w94:T9[])
      n167 = call "IMAQ Overlay ROI"("ROI Descriptor"=w43, "Image"=w74) -> ("Image Out"=→"Right Image 2":T7)  [unwired: 8 in, 1 out]
      n168 = Bundle By Name(cluster="Current Settings", "Range Settings"=w94, "Minimum Match Score"=w97) -> (→"New Settings":T10)
    }
  }
